vi "ROI entry screen-LBox update laser power.vi"(8 "error in (no error)":errorcluster, 11 "Laser Power %":dbl) -> (0 "error out":errorcluster)   [LabVIEW 2020]
uses:
  Typedefs/ROI management FG states.ctl
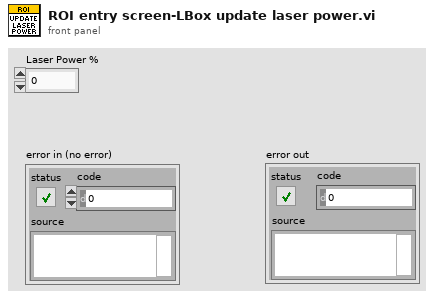
[diagram p1: front panel]
types:
  T1 = typedef "ROI management FG states.ctl" = enum16{"Read", "Write", "Write-from dataset", "Clear Last", "Clear All", "Delete ROI", "Update ROIs time", "Reload last ROI set", "Modify ROI Parameters", "Offset all ROI", "Offset visible ROI", "Modify Dwell Time", "Modify Laser Power"}
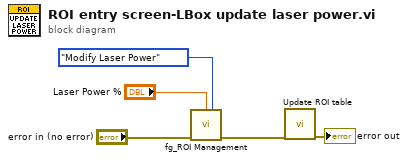
[diagram p0: block diagram]
diagram:
  n1 = call "fg_ROI Management.vi"("Laser Power %"="Laser Power %", "Function"=ROI_management_FG_states."Modify Laser Power", "error in (no error)"="error in (no error)") -> ("error out"=w4:errorcluster)  [unwired: 6 in, 6 out]
  n2 = call "Update ROI table.vi"("error in (no error)"=w4) -> ("error out"=→"error out":errorcluster)  [unwired: 10 in]
